vi "CreatePrivateEvents.vi"(8 "error in (no error)":errorcluster, 11 "CircularBuffer":refnum<class "CircularBuffer.lvclass">) -> (0 "error out":errorcluster, 3 "CircularBuffer out":refnum<class "CircularBuffer.lvclass">)   [LabVIEW 2016, in "CircularBuffer.lvclass"]
doc: "JKI State Machine Objects (SMO) 1.0.2.13\nJKI - JKI\nCopyright (c) 2016, JKI"
uses:
  CircularBuffer.lvclass
  CircularBuffer.lvclass/CircularBuffer.ctl
  Typedefs/NewBufferSize--Cluster.ctl
  Typedefs/PrivateEvents--CircularBuffer.GetElement.ctl
  Typedefs/PrivateEvents--CircularBuffer.Initialize.ctl
  <vilib>/JKI/JKI SMO/SMO/SMO.lvclass
panel:
  # "For instructions on how to use the JKI State Machine Objects, examples and video tutorials, visit:\nhttp://jki.net/state-machine-objects/\n\nJKI State Machine Objects™\nhttp://jki.net/state-machine-objects/\nCopyright (C) 2005-2015, JKI <info@jki.net>\nALL RIGHTS RESERVED"
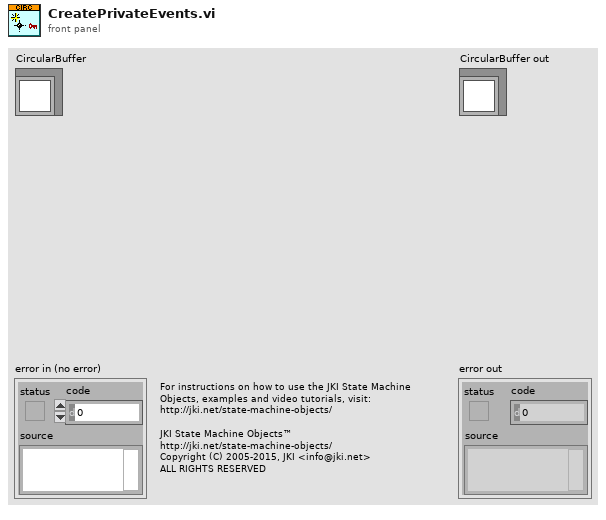
[diagram p1: front panel]
types:
  T1 = typedef "CircularBuffer.lvclass/PrivateData--Ref.ctl" = refnum<data-value>
  T2 = typedef "CircularBuffer.lvclass/PrivateEvents--CircularBuffer.Initialize.ctl" = bool
  T3 = typedef "CircularBuffer.lvclass/PrivateEvents--CircularBuffer.GetElement.ctl" = u32
  T4 = typedef "CircularBuffer.lvclass/NewBufferSize--Cluster.ctl" = cluster{"BufferSize":i32}
  T5 = typedef "CircularBuffer.lvclass/PrivateData--Cluster.ctl" = cluster{"Public Events":T6, "Protected Events":T7, "Private Events":T8, "BufferSize":i32, "CurrentElement":i32, "Elements":refnum<data-value>[], "type":refnum<class "type.lvclass">}
  T6 = typedef "CircularBuffer.lvclass/PublicEvents--Cluster.ctl" = cluster{"Buffer Resize Event":refnum<user-event>}
  T7 = typedef "CircularBuffer.lvclass/ProtectedEvents--Cluster.ctl" = cluster{"placeholder":refnum<user-event>}
  T8 = typedef "CircularBuffer.lvclass/PrivateEvents--Cluster.ctl" = cluster{"New Value":refnum<user-event>, "GetElement":refnum<user-event>, "Initialize":refnum<user-event>}
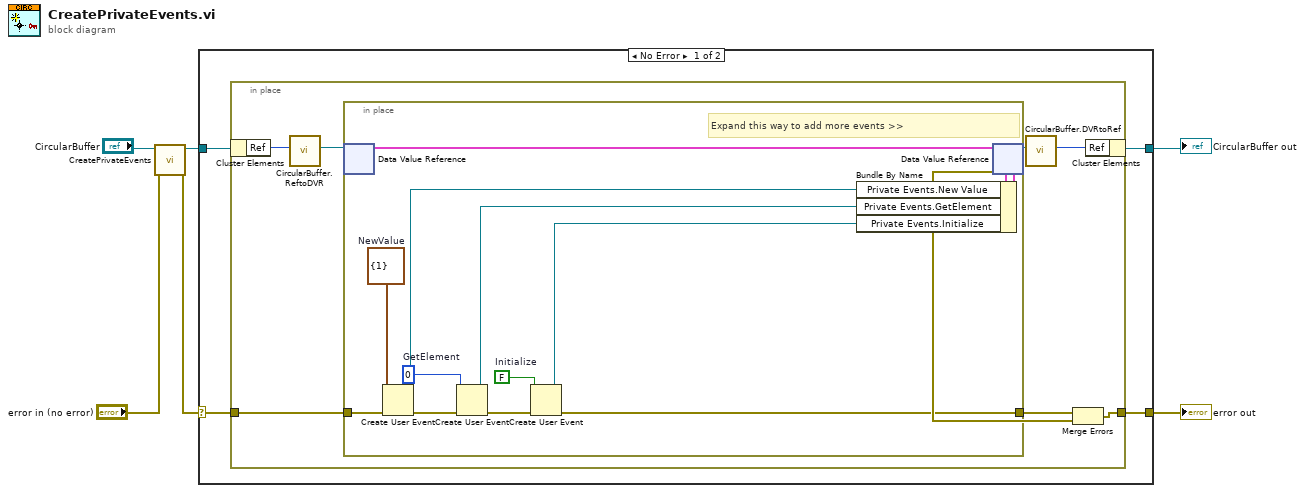
[diagram p0: block diagram]
diagram:
  n1 = call-parent "CreatePrivateEvents.vi"("error in (no error)"="error in (no error)", "SMO"="CircularBuffer") -> ("error out"=w5:errorcluster, "SMO out"=w6:refnum<class "CircularBuffer.lvclass">)  [unwired: 8 in]
  n2 = case shown="No Error" w5 {
    selector: w5 -> [w8 w32]
    tunnel: [w7 w32] -> w1
    tunnel: [w9 w31] -> w3
    tunnel: w6 -> [w10 w31]
    frame No Error {
      n3 = in-place {
        in-place-border: w8 -> [w18]
        in-place-border: [w15] -> w7
        n4 = in-place-cluster #1(w10) -> ("Ref"=w14:u32)
        n5 = call "CircularBuffer.ReftoDVR.vi"("Ref"=w14) -> ("Ref"=w13:T1)  [unwired: 10 in]
        n6 = in-place {
          in-place-border: w18 -> [w28]
          in-place-border: [w21] -> w17
          w20 = T2 FALSE  # Initialize
          w23 = T3 0  # GetElement
          w25 = T4 {"BufferSize"=1}  # NewValue
          # "Expand this way to add more events >>"
          n7 = in-place-dvr #2(w13) -> (w27:T5)  [unwired: 1 out]
          n8 = Create User Event(user event datatype=w25, error in=w28) -> (user event=w26:refnum<user-event>, error out=w29:errorcluster)
          n9 = Create User Event(user event datatype=w23, error in=w29) -> (user event=w22:refnum<user-event>, error out=w24:errorcluster)
          n10 = Create User Event(user event datatype=w20, error in=w24) -> (user event=w19:refnum<user-event>, error out=w21:errorcluster)
          n11 = Bundle By Name(cluster=w27, "Private Events.New Value"=w26, "Private Events.GetElement"=w22, "Private Events.Initialize"=w19) -> (w30:T5)
          n12 = in-place-dvr #2(w30) -> (w12:T1, w16:errorcluster)
        }
        n13 = call "CircularBuffer.DVRtoRef.vi"("Ref"=w12) -> ("Ref"=w11:u32)  [unwired: 10 in]
        n14 = Merge Errors(w17, w16) -> (w15:errorcluster)
        n15 = in-place-cluster #1("Ref"=w11) -> (w9:refnum<class "CircularBuffer.lvclass">)
      }
    }
    frame Error {
    }
  }
  "error out" <- w1
  "CircularBuffer out" <- w3
